vi "OFBS_train_SVM.vi"(6 "Train Data":T5, 8 "error in (no error)":errorcluster, 9 "Nu":dbl, 10 "Parameters":i32[](array[numeric]), 11 "OFBS class in":refnum<class "OptFreqBandsSearch.lvclass">) -> (0 "error out":errorcluster, 1 "Training Results":T1[](array[typedef]) {"Standard Deviation" format="%.2f"}, 2 "Classifier Session (out)":T2, 3 "OFBS class out":refnum<class "OptFreqBandsSearch.lvclass">)   [LabVIEW 2016, in "Optimal Frequency Bands Search.lvlib" / "OptFreqBandsSearch.lvclass"]
doc: "Метод, реализующий построение классификатора на основе многослойного персептрона. Для обучения классификатора используются обучающие данные."
uses:
  OptFreqBandsSearch.lvclass
  OFBS_DataTypes.ctl
  <vilib>/vision/Classification.llb/IMAQ SVM Kernel Options.ctl
  <vilib>/vision/Classification.llb/IMAQ SVM Model Options.ctl
  <vilib>/vision/Classification.llb/IMAQ Classifier Session.ctl
  <vilib>/vision/Classification.llb/IMAQ Classifier SVM Training Results.ctl
  OptFreqBandsSearch.lvclass/OptFreqBandsSearch.ctl
  Optimal Frequency Bands Search.lvlib
  <vilib>/vision/NI_Vision_Development_Module.lvlib
panel:
  in  "Model Options":T3={"SVM Model"=enum."nu-SVC", "Tolerance"=0.001, "Max. Iteration"=100000, "Nu"=0.1, "Shrinking"=FALSE, "Cost"=1.0, "Weighted Cost"=[]}
  in  "Kernel Options":T4={"Kernel"=enum."Linear", "Degree"=3, "Gamma"=1.0, "Coefficient"=0.0, "Sigma"=1.0, "Cache(MB)"=100.0}
  # "This VI is a part of BCI Design library, http://www.ru-bci.org \nCopyright © 2020, Sotnikov Peter, All rights reserved. License: GNU GPLv3"
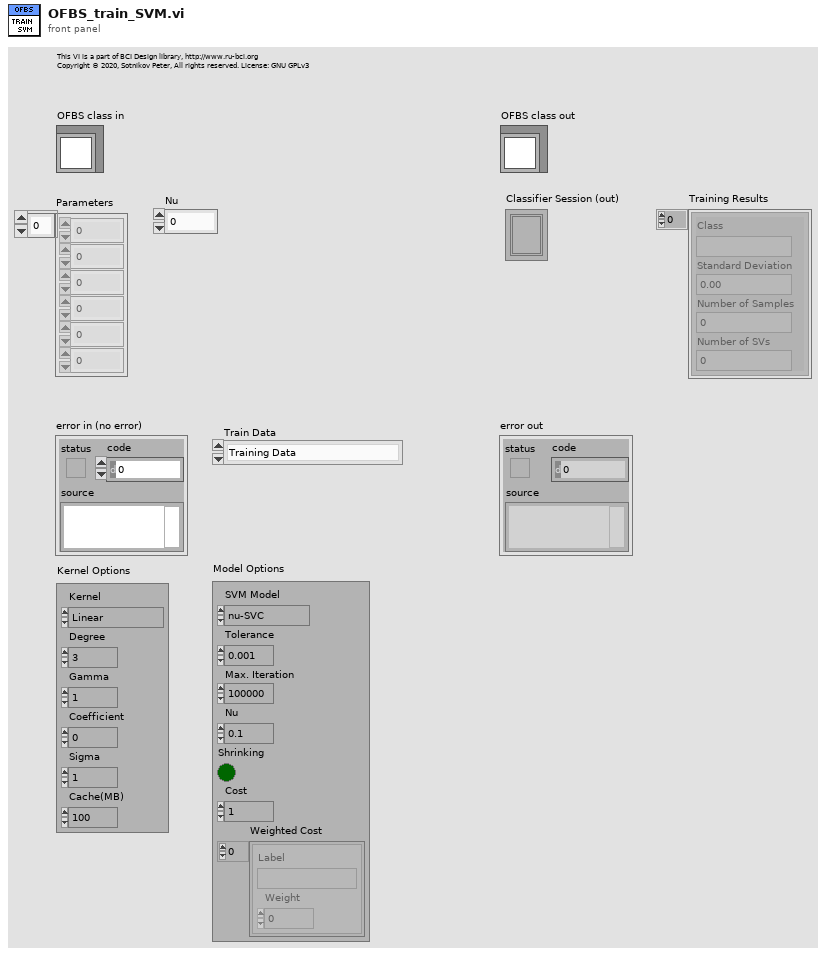
[diagram p1: front panel]
types:
  T1 = typedef "IMAQ Classifier SVM Training Results.ctl" = cluster{"Class":string, "Standard Deviation":sgl, "Number of Samples":i32, "Number of SVs":i32}
  T2 = typedef "IMAQ Classifier Session.ctl" = refnum<k1>
  T3 = typedef "IMAQ SVM Model Options.ctl" = cluster{"SVM Model":enum32{"C-SVC", "nu-SVC", "One Class"}, "Tolerance":dbl, "Max. Iteration":i32, "Nu":dbl, "Shrinking":bool, "Cost":dbl, "Weighted Cost":cluster{"Label":string, "Weight":dbl}[]}
  T4 = typedef "IMAQ SVM Kernel Options.ctl" = cluster{"Kernel":enum32{"Linear", "Polynomial", "Gaussian", "RBF"}, "Degree":i32, "Gamma":dbl, "Coefficient":dbl, "Sigma":dbl, "Cache(MB)":dbl}
  T5 = typedef "Optimal Frequency Bands Search.lvlib/OFBS_DataTypes.ctl" = enum16{"Training Data", "Test Data", "Training Data (cross-check)", "Test Data (cross-check)"}
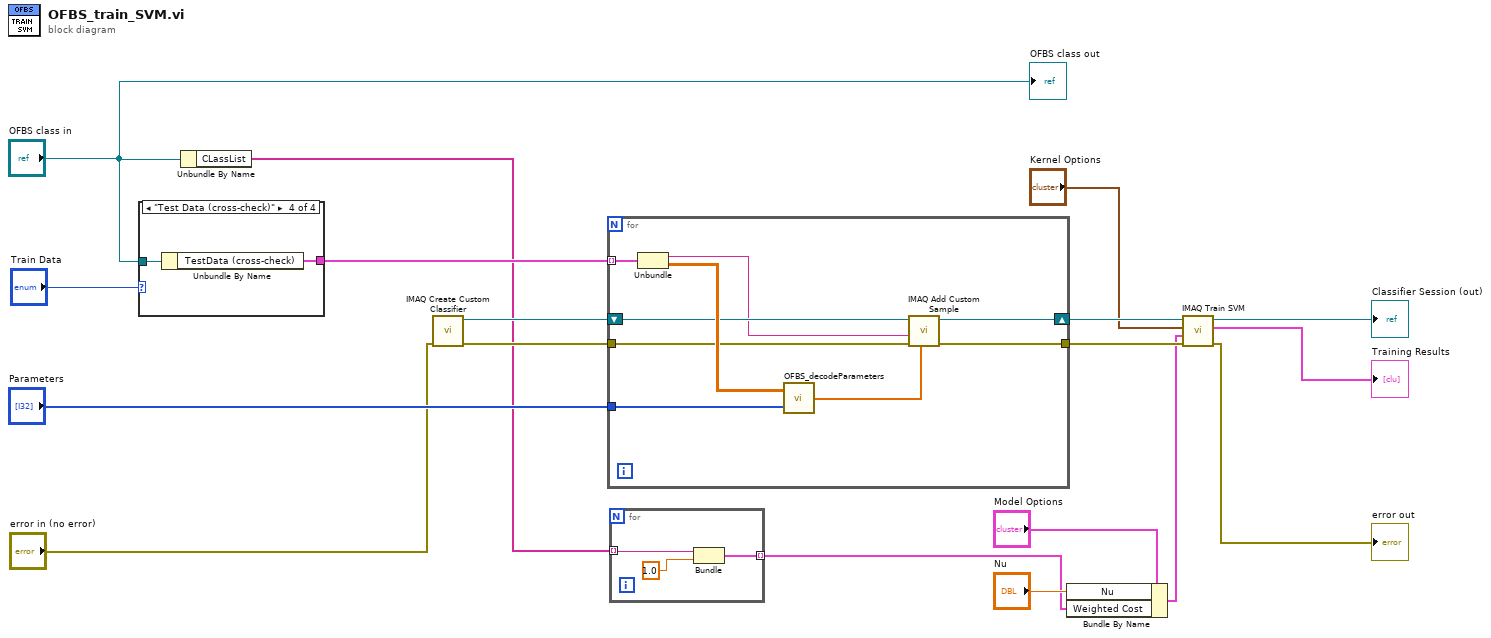
[diagram p0: block diagram]
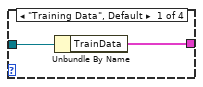
[diagram p2: hidden frame]
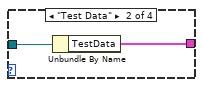
[diagram p3: hidden frame]
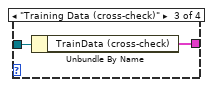
[diagram p4: hidden frame]
diagram:
  n1 = case shown="\"Test Data (cross-check)\"" "Train Data" {
    tunnel: "OFBS class in" -> [w20 w22 w24 w26]
    tunnel: [w19 w21 w23 w25] -> w15
    frame "Training Data", Default {
      n2 = Unbundle By Name(w20) -> ("TrainData"=w19:cluster{"ClassLabel":string, "Trial":dbl[][]}[])
    }
    frame "Test Data" {
      n3 = Unbundle By Name(w22) -> ("TestData"=w21:cluster{"ClassLabel":string, "Trial":dbl[][]}[])
    }
    frame "Training Data (cross-check)" {
      n4 = Unbundle By Name(w24) -> ("TrainData (cross-check)"=w23:cluster{"ClassLabel":string, "Trial":dbl[][]}[])
    }
    frame "Test Data (cross-check)" {
      n5 = Unbundle By Name(w26) -> ("TestData (cross-check)"=w25:cluster{"ClassLabel":string, "Trial":dbl[][]}[])
    }
  }
  n6 = Unbundle By Name("OFBS class in") -> ("CLassList"=w2:string[])
  n7 = call "IMAQ Create Custom Classifier"("error in (no error)"="error in (no error)") -> ("error out"=w11:errorcluster, "Classifier Session"=w14:T2)  [unwired: 9 in]
  n8 = for {
    tunnel: w15 -> [w35] mode=indexing
    tunnel: "Parameters" -> [w33]
    shift-right: [w31] -> w13
    shift-left: w14 -> [w32]
    tunnel: w11 -> [w28]
    tunnel: [w27] -> w10
    n9 = Unbundle(w35) -> ("ClassLabel"=w29:string, "Trial"=w34:dbl[][])
    n10 = call "OFBS_decodeParameters.vi"("Parameters"=w33, "Trial"=w34) -> ("FeatureVector"=w30:dbl[])
    n11 = call "IMAQ Add Custom Sample"("Feature Vector"=w30, "error in (no error)"=w28, "Class"=w29, "Classifier Session"=w32) -> ("error out"=w27:errorcluster, "Classifier Session (dup)"=w31:T2)  [unwired: 6 in]
  }
  n12 = for {
    tunnel: w2 -> [w38] mode=indexing
    tunnel: [w36] -> w1 mode=indexing
    n13 = Bundle("node text"=w38, 1.0) -> (w36:cluster{"node text":string, dbl})  [unwired: 1 in]
  }
  n14 = Bundle By Name(cluster="Model Options", "Nu"="Nu", "Weighted Cost"=w1) -> (w4:T3)
  n15 = call "IMAQ Train SVM"("error in (no error)"=w10, "Model Options"=w4, "Kernel Options"="Kernel Options", "Classifier Session"=w13) -> ("error out"=→"error out":errorcluster, "Training Results"=→"Training Results":T1[], "Classifier Session (dup)"=→"Classifier Session (out)":T2)  [unwired: 4 in, 1 out]
  "OFBS class out" <- "OFBS class in"
